vi "kneighbors.vi"(8 "error in (no error)":errorcluster caption="entrée d'erreur (pas d'erreur)", 11 "KNeighbors.lvclass":refnum<class "KNeighbors.lvclass">) -> (0 "error out":errorcluster caption="sortie d'erreur", 2 "out":T1, 3 "KNeighbors.lvclass 2":refnum<class "KNeighbors.lvclass">)   [LabVIEW 2020, in "KNeighbors.lvclass"]
doc: "Finds the K-neighbors of a point.\n\nReturns indices of and distances to the neighbors of each point.\n\nX : array-like, shape (n_queries, n_features), or (n_queries, n_indexed) if metric == ‘precomputed’, default=None\nThe query point or points. If not provided, neighbors of each indexed point are returned. In this case, the query point is not considered its own neighbor.\n\nn_neighbors : int, default=None\nNumber of neighbors required for each sample. The default is the value passed to the constructor.\n\nreturn_distance : bool, default=True\nWhether or not to return the distances."
uses:
  KNeighbors.lvclass
  C:/Users/cipop/TDF Dropbox/2_Technologies de France/1 - Services et Etudes/PLAIY/2 - DEV/PLAIYLAB/code/Python/Python.lvclass
  C:/Users/cipop/TDF Dropbox/2_Technologies de France/1 - Services et Etudes/PLAIY/2 - DEV/PLAIYLAB/code/Model/Model.lvclass
  C:/Users/cipop/TDF Dropbox/2_Technologies de France/1 - Services et Etudes/PLAIY/2 - DEV/PLAIYLAB/code/Model/Supervised/Neighbors/Neighbors.lvclass
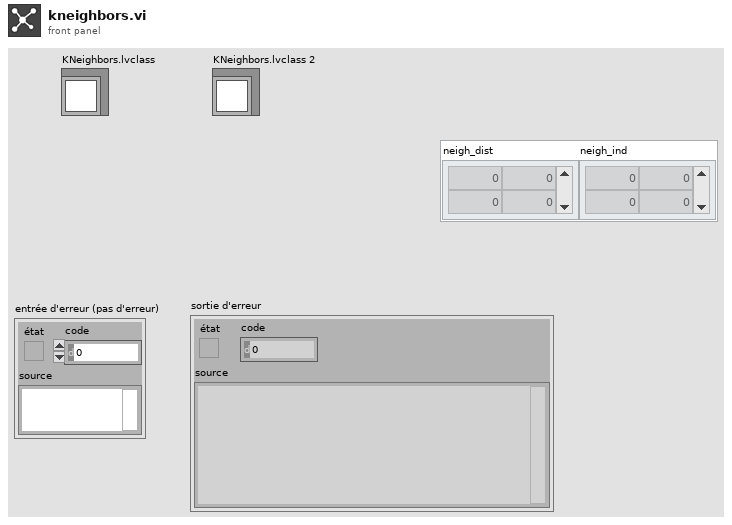
[diagram p1: front panel]
types:
  T1 = cluster{"neigh_dist":dbl[][], "neigh_ind":dbl[][]}
  T2 = typedef "data.ctl" = cluster{"name":string, "X":dbl[][]}
  T3 = typedef "neighbors_data.ctl" = cluster{"y":dbl[][], "sample_weight":dbl[]}
  T4 = typedef "kneighbors_data.ctl" = cluster{"n_neighbors":dbl, "mode":string, "return_distance":bool}
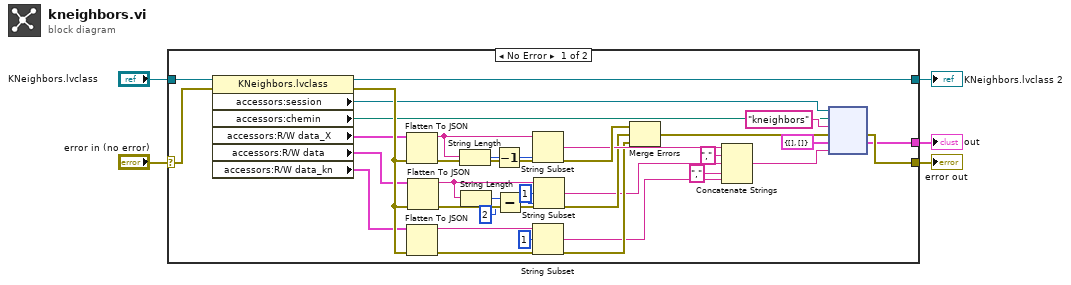
[diagram p0: block diagram]
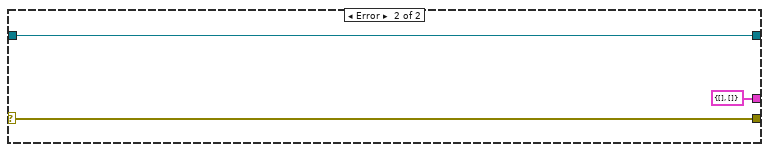
[diagram p2: hidden frame]
diagram:
  n1 = case shown="No Error" "error in (no error)" {
    selector: "error in (no error)" -> [w36 w41]
    tunnel: [w37 w41] -> w2
    tunnel: [w6 w40] -> w3
    tunnel: "KNeighbors.lvclass" -> [w35 w40]
    tunnel: [w24 T1 {"neigh_dist"=[], "neigh_ind"=[]} ("out")] -> w1
    frame No Error {
      n2 = property class="KNeighbors.lvclass"(reference=w35, error in=w36) -> (reference out=w6:refnum<class "KNeighbors.lvclass">, error out=w22:errorcluster, "accessors:session"=w9:refnum<k35>, "accessors:chemin"=w8:path, "accessors:R/W data_X"=w11:T2, "accessors:R/W data"=w10:T3, "accessors:R/W data_kn"=w14:T4)
      n3 = Flatten To JSON(anything=w11, error in (no error)=w22) -> (JSON string=w32:string, 11:w29:errorcluster)  [unwired: 1 in]
      n4 = Flatten To JSON(anything=w14, error in (no error)=w22) -> (JSON string=w30:string, 11:w20:errorcluster)  [unwired: 1 in]
      n5 = Flatten To JSON(anything=w10, error in (no error)=w22) -> (JSON string=w18:string, 11:w19:errorcluster)  [unwired: 1 in]
      n6 = String Length(string=w32) -> (length=w34:i32)
      n7 = String Length(string=w18) -> (length=w13:i32)
      n8 = Decrement(x=w34) -> (x-1=w33:i32)
      n9 = Subtract(x=w13, y=2) -> (x-y=w23:i32)
      n10 = String Subset(string=w32, length (rest)=w33) -> (substring=w27:string)  [unwired: 1 in]
      n11 = String Subset(string=w30, offset (0)=1) -> (substring=w15:string)  [unwired: 1 in]
      n12 = String Subset(string=w18, offset (0)=1, length (rest)=w23) -> (substring=w17:string)
      n13 = Merge Errors(w29, w19, w20) -> (w7:errorcluster)
      n14 = Concatenate Strings(w27, "," ("string"), w17, "," ("string"), w15) -> (w26:string)
      n15 = node(w9, w8, "kneighbors" ("nom de la fonction"), w7, T1 {"neigh_dist"=[], "neigh_ind"=[]} ("out"), w26) -> (w37:errorcluster, w24:T1)  [unwired: 1 in, 3 out]
    }
    frame Error {
    }
  }
  "error out" <- w2
  "KNeighbors.lvclass 2" <- w3
  "out" <- w1
